vi "Test.vi"() -> ()   [LabVIEW 2016]
panel:
  in  "Boolean 2":bool=TRUE
  in  "Boolean":bool
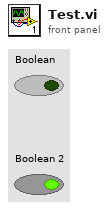
[diagram p1: front panel]
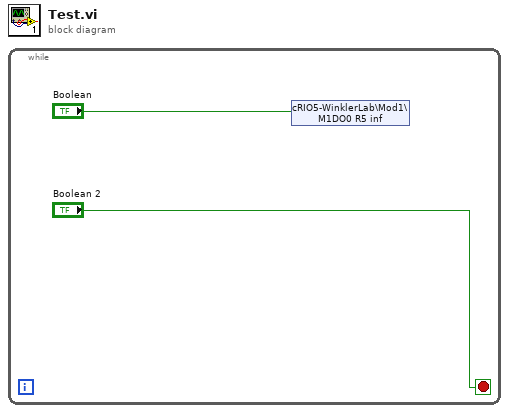
[diagram p0: block diagram]
diagram:
  n1 = while {
    stop <- "Boolean 2" stop-if-true
    n2 = shared-variable "cRIO5-WinklerLab\\Mod1\\M1DO0 R5 inf"("Boolean") -> ()  [unwired: 1 in, 1 out]
  }
